vi "GotoWaypoint.vi"(0 "MDF In":T2(array[cluster]), 1 "WhereAmI? Clean":T3, 2 "XPriorIn":dbl, 3 "YPriorIn":dbl, 4 "WhatAroundMe? Clean":cluster{"T":dbl, "Range":dbl, "Bearing":dbl}[](array[cluster]), 5 "CurrentSteerAngle":dbl, 6 "InhibitIn":bool) -> (7 "SteerAngle":dbl, 12 "Vel":dbl, 13 "InhibitOut":bool, 15 "ActCommand":dbl[](array[numeric]), 16 "XPriorOut":dbl, 17 "YPriorOut":dbl, 18 "MDF Out":T2(array[cluster]), 19 "BehCom":T1(ring))   [LabVIEW 2012]
doc: "This subVI contains the Forebrain Goto Waypoint behaviors. Its inputs are the outputs of thewhat and where SENSE processes, theMission efinition Filet, a suppression value from another co-brahvior and an inhibit signal to turn the behavior off. The outputs are a 90 element steering array and a suppression value to diminish the output of co-behaviors.\n\nIt is designed to work with a 90 element behavior arbiter."
uses:
  <vilib>/Analysis/1siggen.llb/Ramp Pattern by Samples.vi
  <vilib>/gmath/statdist.llb/Normal PDF.vi
  <vilib>/gmath/NI_Gmath.lvlib
  <vilib>/Analysis/NI_AALBase.lvlib
panel:
  out "loop index":i32
  in  "HowAmI? Clean":cluster{"T":dbl, "Battery":dbl, "Temp":dbl}
  # "This VI contains the go to waypoint behavior  at the Forebrain level"
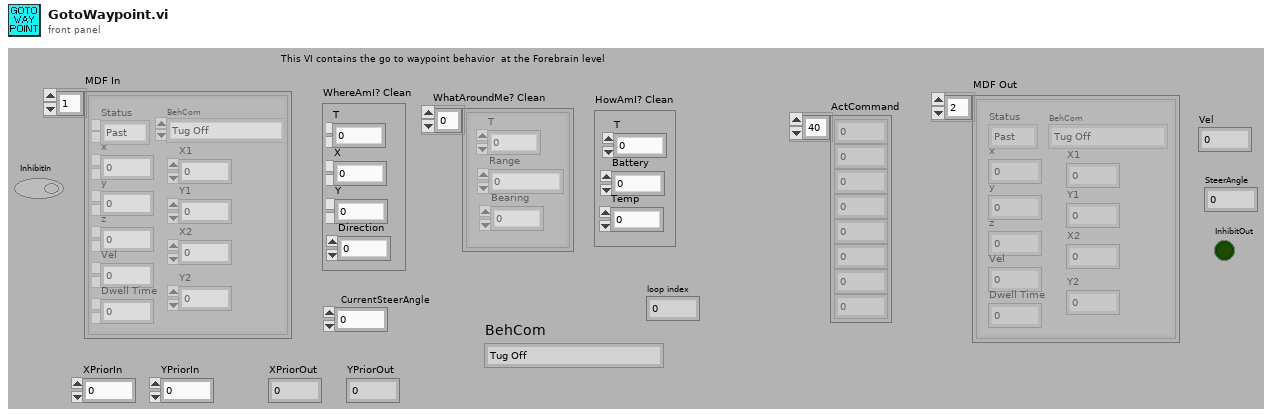
[diagram p1: front panel]
types:
  T1 = enum16{"Tug Off", "Manual Mode", "Goto WayPoint", "Back Up", "Circle", "Left Wall Follow", "Right Wall Follow", "Hunt"}
  T2 = cluster{"Status":enum16{"Past", "Current", "Future"}, "x":dbl, "y":dbl, "z":dbl, "Vel":dbl, "Dwell Time":dbl, "BehCom":enum16{"Tug Off", "Manual Mode", "Goto WayPoint", "Back Up", "Gate", "Left Wall Follow", "Right Wall Follow", "Hunt"}, "X1":dbl, "Y1":dbl, "X2":dbl, "Y2":dbl}[]
  T3 = cluster{"T":dbl, "X":dbl, "Y":dbl, "Direction":dbl}
  T4 = enum16{"Tug Off", "Manual Mode", "Goto WayPoint", "Back Up", "Gate", "Left Wall Follow", "Right Wall Follow", "Hunt"}
  T5 = cluster{"Status":enum16{"Past", "Current", "Future"}, "x":dbl, "y":dbl, "z":dbl, "Vel":dbl, "Dwell Time":dbl, "BehCom":enum16{"Tug Off", "Manual Mode", "Goto WayPoint", "Back Up", "Gate", "Left Wall Follow", "Right Wall Follow", "Hunt"}, "X1":dbl, "Y1":dbl, "X2":dbl, "Y2":dbl}
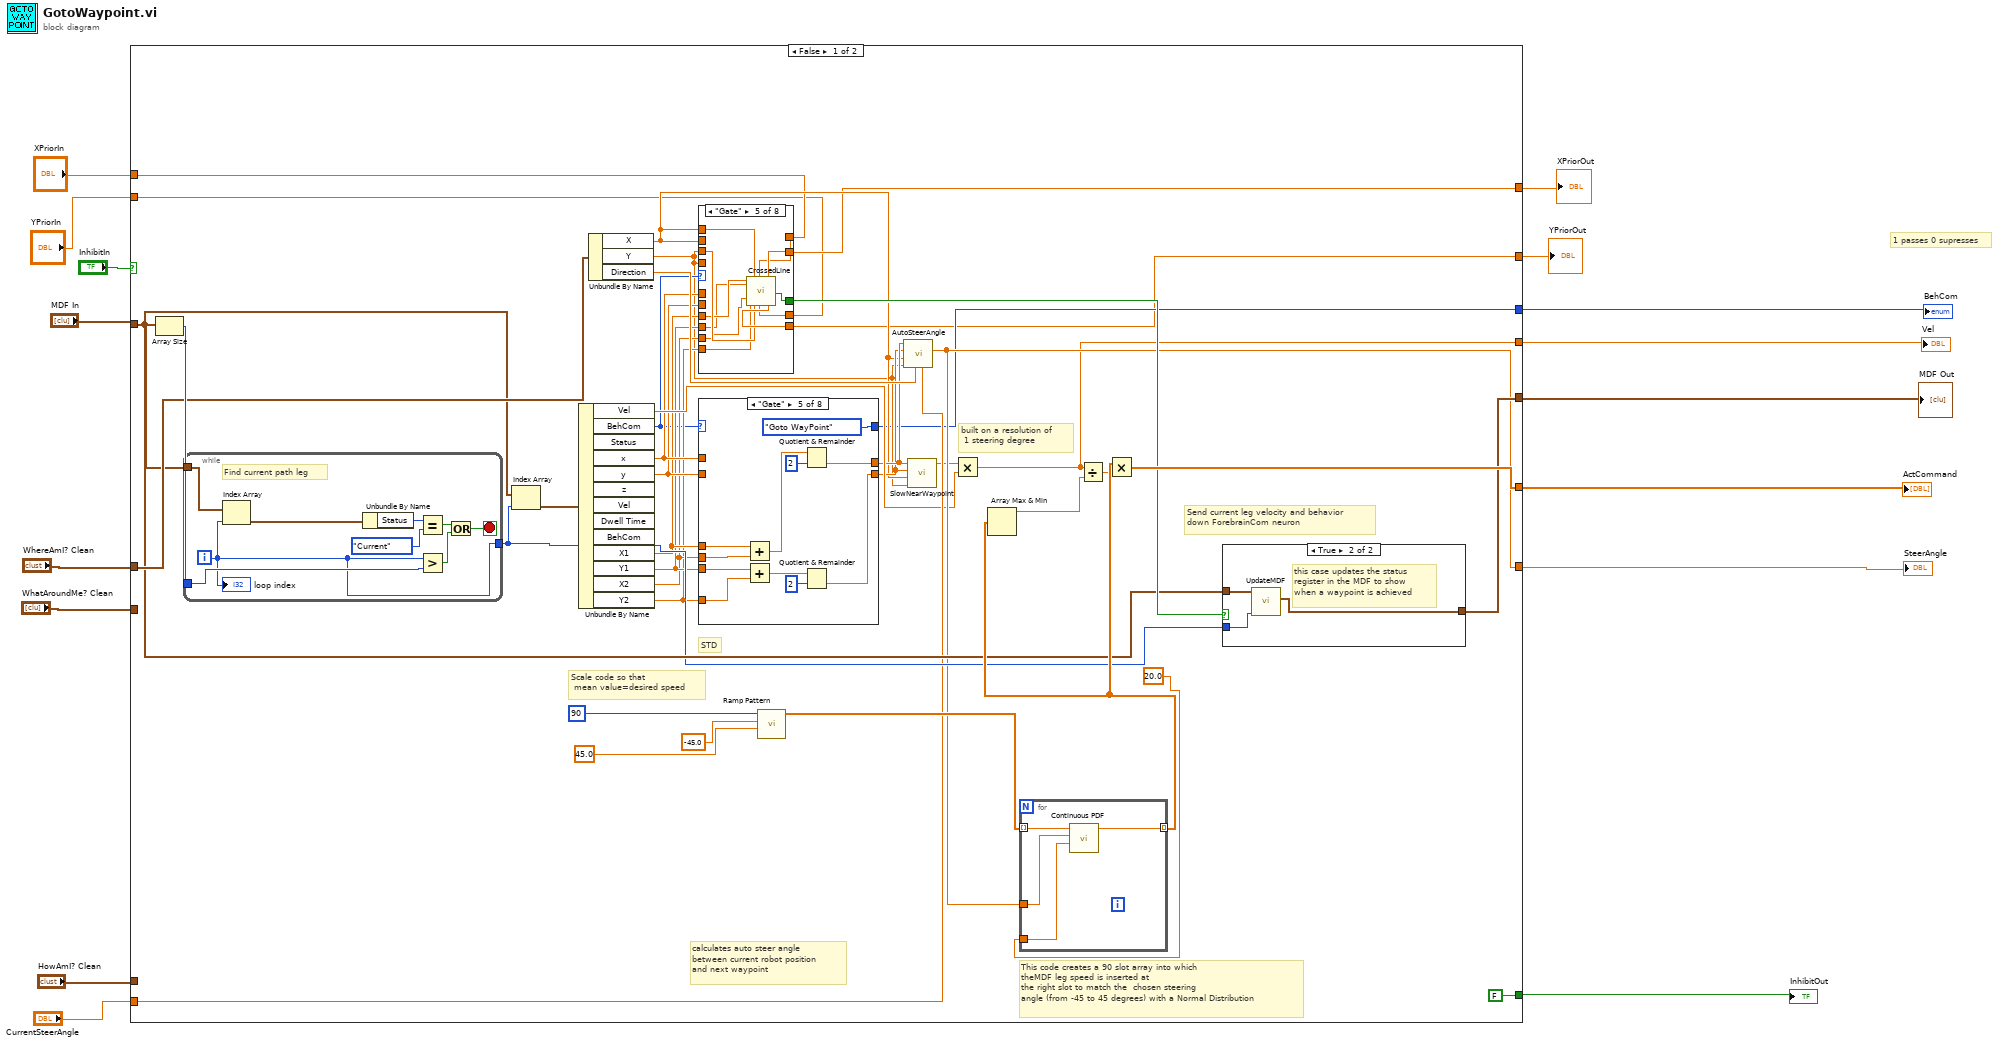
[diagram p0: block diagram]
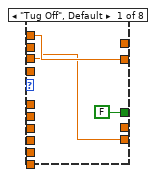
[diagram p9: hidden frame]
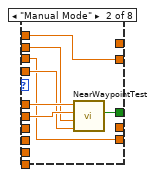
[diagram p10: hidden frame]
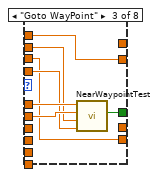
[diagram p11: hidden frame]
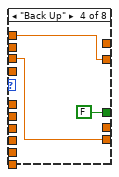
[diagram p12: hidden frame]
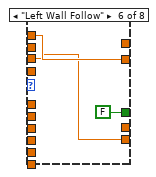
[diagram p13: hidden frame]
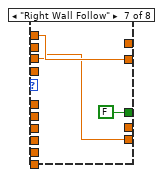
[diagram p14: hidden frame]
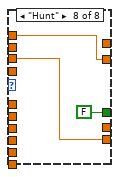
[diagram p15: hidden frame]
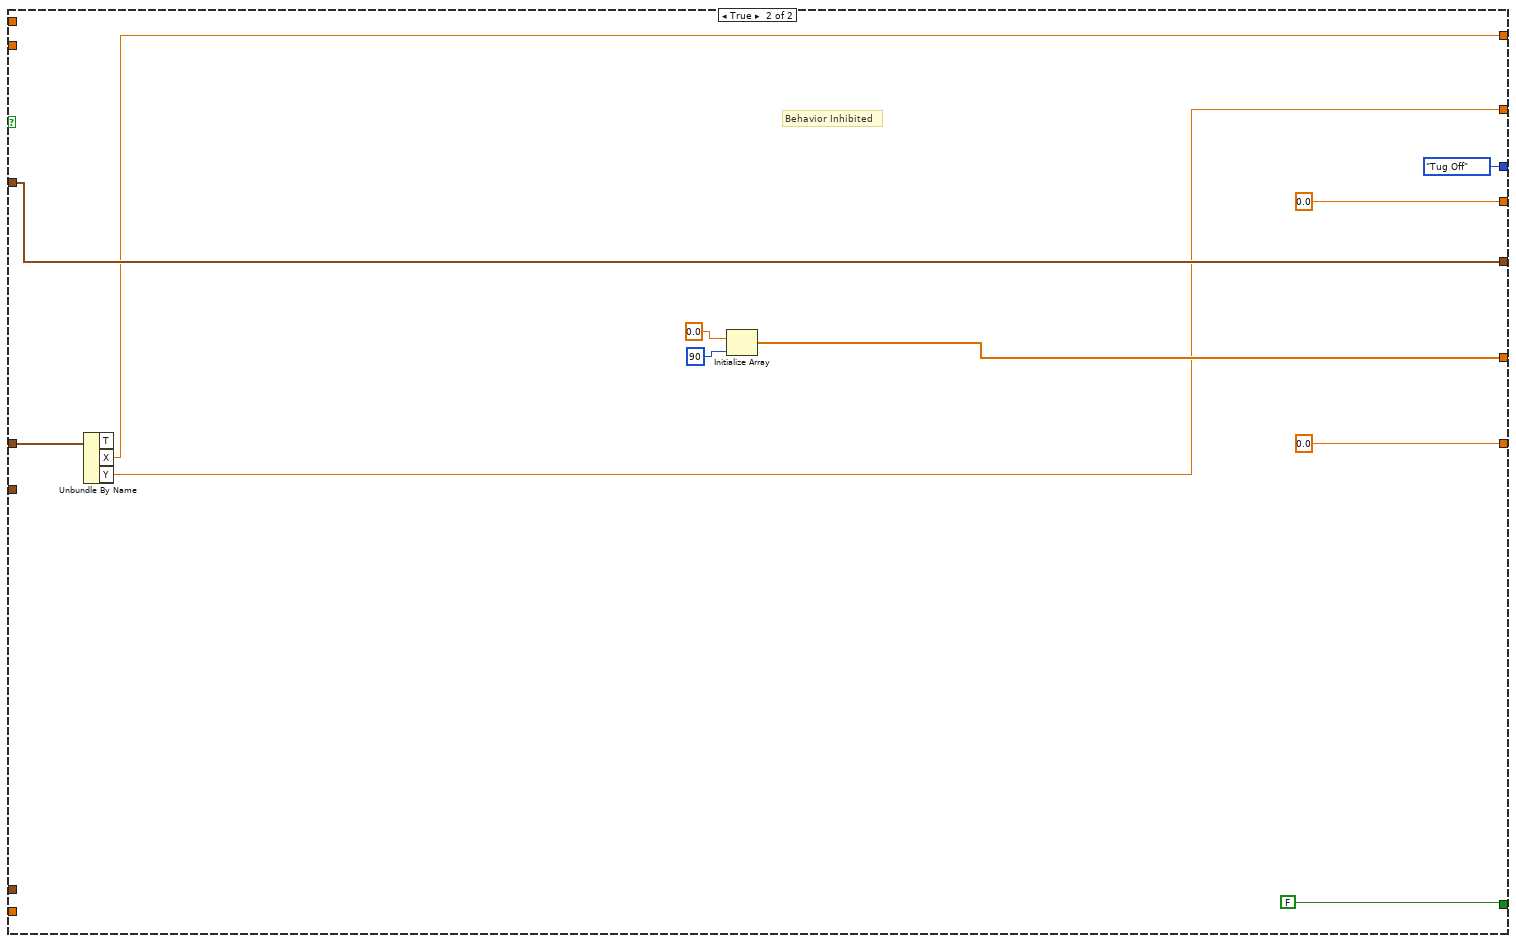
[diagram p17: hidden frame]
diagram:
  # "1 passes 0 supresses"
  n1 = case shown="False" "InhibitIn" {
    tunnel: "WhatAroundMe? Clean" -> [_ _]
    tunnel: "WhereAmI? Clean" -> [w53 w147]
    tunnel: "HowAmI? Clean" -> [_ _]
    tunnel: [w43 w154] -> w12
    tunnel: [FALSE ("InhibitOut") FALSE ("InhibitOut")] -> w5
    tunnel: "MDF In" -> [w40 w151]
    tunnel: [w39 w151] -> w10
    tunnel: [w34 0.0 ("Vel")] -> w9
    tunnel: [w37 0.0 ("SteerAngle")] -> w8
    tunnel: "CurrentSteerAngle" -> [w36 _]
    tunnel: [w21 T1."Tug Off" ("BehCom")] -> w6
    tunnel: [w20 w145] -> w4
    tunnel: [w19 w146] -> w3
    tunnel: "XPriorIn" -> [w18 _]
    tunnel: "YPriorIn" -> [w17 _]
    frame False {
      # "Send current leg velocity and behavior\ndown ForebrainCom neuron"
      # "calculates auto steer angle\nbetween current robot position\nand next waypoint"
      # "built on a resolution of\n 1 steering degree"
      # "Scale code so that\n mean value=desired speed"
      # "STD"
      # "This code creates a 90 slot array into which\ntheMDF leg speed is inserted at\nthe right slot to match the  chosen steering\nangle (from -45 to 45 degrees) with a Normal Distribution"
      n2 = Array Size(array=w40) -> (size(s)=w54:i32)
      n3 = while {
        tunnel: w54 -> [w144]
        tunnel: w40 -> [w141]
        tunnel: [w136] -> w38
        i -> [w136]
        stop <- w143 stop-if-true
        # "Find current path leg"
        n4 = Index Array "Index Array"(array=w141, index=w136) -> (element=w138:T5)
        n5 = Unbundle By Name(w138) -> ("Status"=w139:enum16{"Past", "Current", "Future"})
        n6 = Equal?(x=w139, y=enum16{"Past", "Current", "Future"}."Current") -> (x = y?=w140:bool)
        n7 = Greater?(x=w136, y=w144) -> (0:w142:bool)
        n8 = Or(x=w140, y=w142) -> (x .or. y?=w143:bool)
        "loop index" <- w136
      }
      n9 = Index Array "Index Array"(array=w40, index=w38) -> (element=w52:T5)
      n10 = Unbundle By Name(w52) -> ("Vel"=w35:dbl, "BehCom"=w26:T4, "x"=w32:dbl, "y"=w31:dbl, "X1"=w30:dbl, "Y1"=w29:dbl, "X2"=w28:dbl, "Y2"=w27:dbl)  [unwired: 5 out]
      n11 = Unbundle By Name(w53) -> ("X"=w23:dbl, "Y"=w22:dbl, "Direction"=w42:dbl)
      n12 = case shown="\"Gate\"" w26 {
        tunnel: [FALSE w97 w104 FALSE w118 FALSE FALSE FALSE] -> w41
        tunnel: w32 -> [_ w96 w103 _ _ _ _ _]
        tunnel: w31 -> [_ w95 w102 _ _ _ _ _]
        tunnel: w23 -> [_ w94 w101 _ _ _ _ _]
        tunnel: w22 -> [_ w93 w100 _ _ _ _ _]
        tunnel: w30 -> [_ _ _ _ w113 _ _ _]
        tunnel: w29 -> [_ _ _ _ w112 _ _ _]
        tunnel: w28 -> [_ _ _ _ w111 _ _ _]
        tunnel: w27 -> [_ _ _ _ w110 _ _ _]
        tunnel: w23 -> [w89 w92 w99 w106 w115 w120 w123 w125]
        tunnel: w22 -> [w88 w91 w98 w105 w114 w119 w122 w126]
        tunnel: [w88 w91 w98 w105 w117 w119 w122 w126] -> w20
        tunnel: [w89 w92 w99 w106 w116 w120 w123 w125] -> w19
        tunnel: w18 -> [_ _ _ _ w109 _ _ _]
        tunnel: w17 -> [_ _ _ _ w108 _ _ _]
        frame "Tug Off", Default {
        }
        frame "Manual Mode" {
          n13 = call "NearWaypointTest.vi"("Yrobot"=w93, "Xrobot"=w94, "Ywaypoint"=w95, "Xwaypoiny"=w96) -> ("AtWaypoint"=w97:bool)  [unwired: 7 in]
        }
        frame "Goto WayPoint" {
          n14 = call "NearWaypointTest.vi"("Yrobot"=w100, "Xrobot"=w101, "Ywaypoint"=w102, "Xwaypoiny"=w103) -> ("AtWaypoint"=w104:bool)  [unwired: 7 in]
        }
        frame "Back Up" {
        }
        frame "Gate" {
          n15 = call "CrossedLine.vi"("Xpoint1"=w113, "Ypoint1"=w112, "Xpoint2"=w111, "Ypoint2"=w110, "XpointC"=w115, "YpointC"=w114, "XpointP"=w109, "YpointP"=w108) -> ("NextPriorX"=w116:dbl, "NextPriorY"=w117:dbl, "CrossedLine"=w118:bool)  [unwired: 9 in]
        }
        frame "Left Wall Follow" {
        }
        frame "Right Wall Follow" {
        }
        frame "Hunt" {
        }
      }
      n16 = case shown="\"Gate\"" w26 {
        selector: w26 -> [w58 w61 w64 w67 _ w81 w84 w87]
        tunnel: [w58 w61 w64 w67 T4."Goto WayPoint" ("BehCom") w81 w84 w87] -> w21
        tunnel: w32 -> [w56 w59 w63 w65 _ w80 w82 w85]
        tunnel: w31 -> [w57 w60 w62 w66 _ w79 w83 w86]
        tunnel: w30 -> [_ _ _ _ w71 _ _ _]
        tunnel: w29 -> [_ _ _ _ w70 _ _ _]
        tunnel: w28 -> [_ _ _ _ w69 _ _ _]
        tunnel: w27 -> [_ _ _ _ w68 _ _ _]
        tunnel: [w57 w60 w62 w66 w77 w79 w83 w86] -> w24
        tunnel: [w56 w59 w63 w65 w76 w80 w82 w85] -> w25
        frame "Tug Off", Default {
        }
        frame "Manual Mode" {
        }
        frame "Goto WayPoint" {
        }
        frame "Back Up" {
        }
        frame "Gate" {
          n17 = Add(x=w71, y=w69) -> (x+y=w74:dbl)
          n18 = Add(x=w70, y=w68) -> (x+y=w75:dbl)
          n19 = Quotient & Remainder(x=w74, y=2) -> (floor(x/y)=w76:dbl)  [unwired: 1 out]
          n20 = Quotient & Remainder(x=w75, y=2) -> (floor(x/y)=w77:dbl)  [unwired: 1 out]
        }
        frame "Left Wall Follow" {
        }
        frame "Right Wall Follow" {
        }
        frame "Hunt" {
        }
      }
      n21 = call-poly <vilib>:"Ramp Pattern.vi"("start"=45.0, "end"=-45.0 ("end (Normal)"), "samples"=90) -> ("Ramp Pattern"=w46:dbl[])  [unwired: 7 in, 1 out]
      n22 = call "AutoSteerAngle.vi"("CurrentSteerAngle"=w36, "CurrentDirection"=w42, "Ycurrent"=w22, "Xcurrent"=w23, "Ywaypoint"=w24, "Xwaypoint"=w25) -> ("NewSteerAngle"=w37:dbl)  [unwired: 5 in]
      n23 = call "SlowNearWaypoint.vi"("Yrobot"=w22, "Xrobot"=w23, "Ywaypoint"=w24, "Xwaypoiny"=w25) -> ("SpeedDecrease"=w33:dbl)  [unwired: 7 in]
      n24 = Multiply(x=w33, y=w35) -> (x*y=w34:dbl)
      n25 = for {
        tunnel: w46 -> [w135] mode=indexing
        tunnel: 20.0 ("std (Normal)") -> [w134]
        tunnel: [w133] -> w50 mode=indexing
        tunnel: w37 -> [w132]
        n26 = call-poly <vilib>:"Continuous PDF.vi"("std"=w134, "mean"=w132, "x"=w135) -> ("pdf(x)"=w133:dbl)  [unwired: 7 in, 1 out]
      }
      n27 = Array Max & Min(array=w50) -> (max value=w48:dbl)  [unwired: 3 out]
      n28 = Divide(x=w34, y=w48) -> (x/y=w49:dbl)
      n29 = Multiply(x=w50, y=w49) -> (x*y=w43:dbl[])
      n30 = case shown="True" w41 {
        tunnel: w40 -> [w128 w131]
        tunnel: [w128 w129] -> w39
        tunnel: w38 -> [_ w130]
        frame False {
          # "robot not near waypoint\npass MDF through unaltered"
        }
        frame True {
          # "this case updates the status\nregister in the MDF to show \nwhen a waypoint is achieved"
          n31 = call "UpdateMDF.vi"("Index"=w130, "MDF_In"=w131) -> ("MDF_Out"=w129:T2)  [unwired: 9 in]
        }
      }
    }
    frame True {
      # "Behavior Inhibited"
      n32 = Unbundle By Name(w147) -> ("X"=w146:dbl, "Y"=w145:dbl)  [unwired: 1 out]
      n33 = Initialize Array "Initialize Array"(0.0 ("element"), 90 ("dimension size")) -> (w154:dbl[])
    }
  }
  "ActCommand" <- w12
  "InhibitOut" <- w5
  "MDF Out" <- w10
  "Vel" <- w9
  "SteerAngle" <- w8
  "BehCom" <- w6
  "XPriorOut" <- w3
  "YPriorOut" <- w4
